vi "XYGraph - Colors.vi"(8 "error in":errorcluster, 10 "Ctl Refnum":refnum<vi>, 11 "Material-Scheme in":refnum<class "Material-Scheme.lvclass">) -> (0 "error out":errorcluster)   [LabVIEW 2021, in "TSC Material Theme.lvlib" / "Material-Scheme.lvclass"]
doc: "Set the colors for an XY waveform graph type.\n\n<b>Code Developed By:</b>\nTechnology Service Corporation\n1983 S Liberty Drive\nBloomington, IN 47403\nwww.tsc.com/atcs\n\nDeveloper:\nDaniel Coons"
uses:
  Material-Scheme.lvclass
  Material-Scheme.lvclass/Material-Scheme.ctl
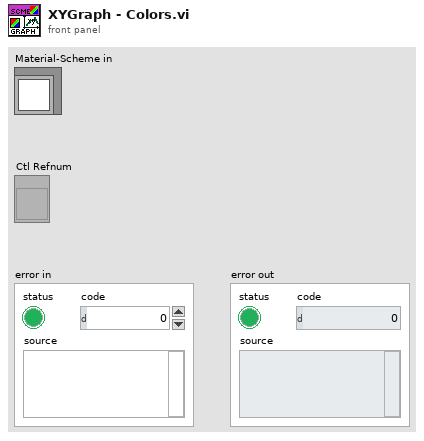
[diagram p1: front panel]
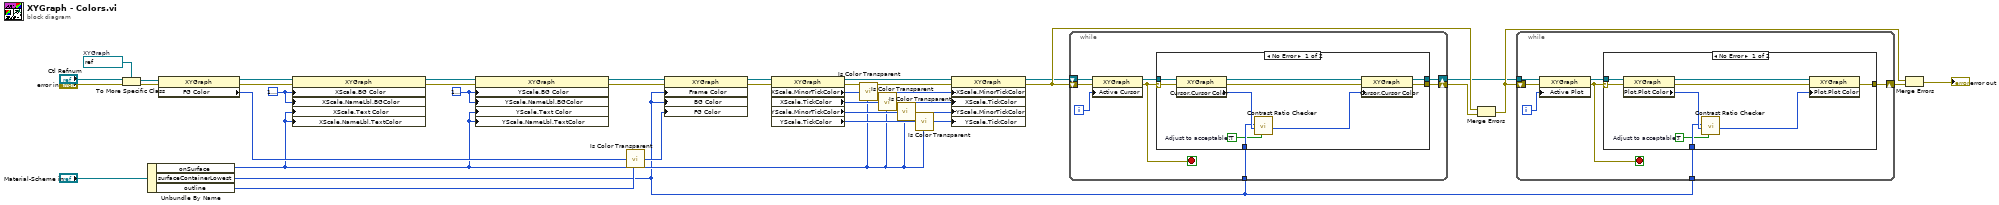
[diagram p0: block diagram]
diagram:
  w21 = u32 16777216 ("X Scale.Name Label.Colors:FG Color")
  w16 = u32 16777216 ("X Scale.Name Label.Colors:FG Color")
  w19 = refnum<vi> refnum  # XYGraph
  n1 = To More Specific Class(target class=w19, reference="Ctl Refnum", error in="error in") -> (specific class reference=w24:refnum<vi>, error out=w37:errorcluster)
  n2 = Unbundle By Name("Material-Scheme in") -> ("onSurface"=w5:u32, "surfaceContainerLowest"=w1:u32, "outline"=w23:u32)
  n3 = property class="XYGraph"(reference=w24, error in=w37) -> (reference out=w25:refnum<vi>, error out=w38:errorcluster, "FG Color"=w26:u32)
  n4 = property class="XYGraph"(reference=w25, error in=w38, "XScale.BG Color"=w16, "XScale.NameLbl.BGColor"=w16, "XScale.Text Color"=w5, "XScale.NameLbl.TextColor"=w5) -> (reference out=w20:refnum<vi>, error out=w35:errorcluster)
  n5 = property class="XYGraph"(reference=w20, error in=w35, "YScale.BG Color"=w21, "YScale.NameLbl.BGColor"=w21, "YScale.Text Color"=w5, "YScale.NameLbl.TextColor"=w5) -> (reference out=w22:refnum<vi>, error out=w36:errorcluster)
  n6 = call "Is Color Transparent.vi"("original color"=w26, "desired color"=w23) -> ("updated color"=w15:u32)  [unwired: 3 in]
  n7 = property class="XYGraph"(reference=w22, error in=w36, "Frame Color"=w1, "BG Color"=w1, "FG Color"=w15) -> (reference out=w14:refnum<vi>, error out=w31:errorcluster)
  n8 = property class="XYGraph"(reference=w14, error in=w31) -> (reference out=w4:refnum<vi>, error out=w30:errorcluster, "XScale.MinorTickColor"=w13:u32, "XScale.TickColor"=w11:u32, "YScale.MinorTickColor"=w9:u32, "YScale.TickColor"=w7:u32)
  n9 = call "Is Color Transparent.vi"("original color"=w13, "desired color"=w5) -> ("updated color"=w12:u32)  [unwired: 3 in]
  n10 = call "Is Color Transparent.vi"("original color"=w11, "desired color"=w5) -> ("updated color"=w10:u32)  [unwired: 3 in]
  n11 = call "Is Color Transparent.vi"("original color"=w9, "desired color"=w5) -> ("updated color"=w8:u32)  [unwired: 3 in]
  n12 = call "Is Color Transparent.vi"("original color"=w7, "desired color"=w5) -> ("updated color"=w6:u32)  [unwired: 3 in]
  n13 = property class="XYGraph"(reference=w4, error in=w30, "XScale.MinorTickColor"=w12, "XScale.TickColor"=w10, "YScale.MinorTickColor"=w8, "YScale.TickColor"=w6) -> (reference out=w3:refnum<vi>, error out=w28:errorcluster)
  n14 = while {
    shift-right: [w44] -> w27
    shift-left: w28 -> [w46]
    tunnel: w1 -> [w41]
    shift-right: [w39] -> w2
    shift-left: w3 -> [w40]
    i -> [w43]
    stop <- w45 stop-if-true
    n15 = property class="XYGraph"(reference=w40, error in=w46, "Active Cursor"=w43) -> (reference out=w42:refnum<vi>, error out=w45:errorcluster)
    n16 = case shown="No Error" w45 {
      selector: w45 -> [w56 _]
      tunnel: [w54 _] -> w44
      tunnel: w42 -> [w53 w57]
      tunnel: w41 -> [w51 _]
      tunnel: [w47 w57] -> w39
      frame No Error {
        w50 = TRUE  # Adjust to acceptable?
        n17 = property class="XYGraph"(reference=w53, error in=w56) -> (reference out=w49:refnum<vi>, error out=w55:errorcluster, "Cursor.Cursor Color"=w52:u32)
        n18 = call "Contrast Ratio Checker.vi"("Adjust to acceptable?"=w50, "On Color"=w52, "Background Color"=w51) -> ("Adjusted Color"=w48:u32)  [unwired: 6 in, 2 out]
        n19 = property class="XYGraph"(reference=w49, error in=w55, "Cursor.Cursor Color"=w48) -> (reference out=w47:refnum<vi>, error out=w54:errorcluster)
      }
      frame Error {
      }
    }
  }
  n20 = Merge Errors(w28, w27) -> (w29:errorcluster)
  n21 = while {
    shift-right: [w62] -> w33
    shift-left: w29 -> [w64]
    tunnel: w1 -> [w59]
    tunnel: w2 -> [w58]
    i -> [w61]
    stop <- w63 stop-if-true
    n22 = property class="XYGraph"(reference=w58, error in=w64, "Active Plot"=w61) -> (reference out=w60:refnum<vi>, error out=w63:errorcluster)
    n23 = case shown="No Error" w63 {
      selector: w63 -> [w73 _]
      tunnel: [w71 _] -> w62
      tunnel: w60 -> [w70 _]
      tunnel: w59 -> [w68 _]
      frame No Error {
        w67 = TRUE  # Adjust to acceptable?
        n24 = property class="XYGraph"(reference=w70, error in=w73) -> (reference out=w66:refnum<vi>, error out=w72:errorcluster, "Plot.Plot Color"=w69:u32)
        n25 = call "Contrast Ratio Checker.vi"("Adjust to acceptable?"=w67, "On Color"=w69, "Background Color"=w68) -> ("Adjusted Color"=w65:u32)  [unwired: 6 in, 2 out]
        n26 = property class="XYGraph"(reference=w66, error in=w72, "Plot.Plot Color"=w65) -> (error out=w71:errorcluster)  [unwired: 1 out]
      }
      frame Error {
      }
    }
  }
  n27 = Merge Errors(w29, w33) -> (→"error out":errorcluster)
